vi "Second Subpanel.vi"() -> ()   [LabVIEW 2015]
panel:
  in  "stop":bool
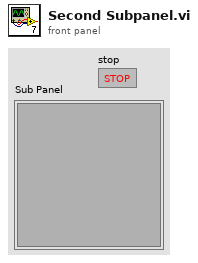
[diagram p1: front panel]
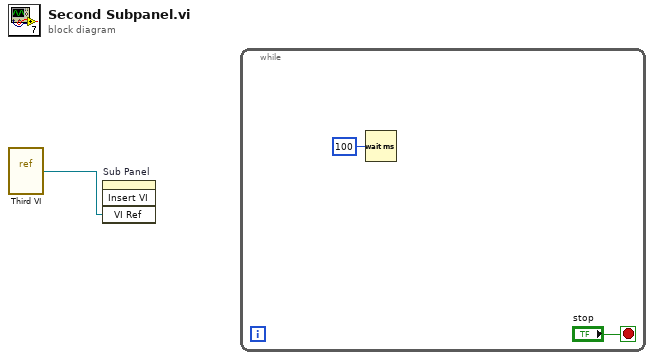
[diagram p0: block diagram]
diagram:
  n1 = vi-ref "Third VI.vi"() -> (w1:refnum<vi>)
  n2 = invoke on="Sub Panel" class="SubPnl" method="Insert VI"("VI Ref"=w1) -> ()  [unwired: 3 in, 4 out]
  n3 = while {
    stop <- "stop" stop-if-true
    n4 = Wait (ms)(milliseconds to wait=u32 100) -> ()  [unwired: 1 out]
  }
